vi "TX-SIS-BPCS-Modbus.vi"() -> ()   [LabVIEW 2018]
uses:
  <vilib>/Platform/TimedLoop/XDataNode/timing_clust.ctl
  <vilib>/Platform/TimedLoop/XDataNode/nitl_modes.ctl
  <vilib>/Platform/TimedLoop/XDataNode/wakeup.ctl
  <vilib>/Modbus/slave/Create Slave Instance (TCP).vi
  Global Variables.vi
  <vilib>/Modbus/slave/Modbus Slave.lvclass
  <vilib>/Platform/TimedLoop/XDataNode/XDataNode.xnode
  <vilib>/Platform/TimedLoop/XDataNode/XDNodeRunTimeDep.lvlib
panel:
  out "TX-SIS-BPCS-Array":bool[](array[boolean])
  in  "stop":bool
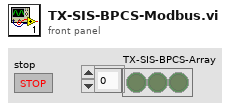
[diagram p1: front panel]
types:
  T1 = typedef "XDNodeRunTimeDep.lvlib/timing_clust.ctl" = cluster{"Expected End [f-1]":u64, "Actual End [f-1]":u64, "Finished Late? [f-1]":bool, "Expected End [i-1]":u64, "Actual End [i-1]":u64, "Finished Late? [i-1]":bool, "Expected Start [i]":u64, "Actual Start [i]":u64, "Expected Start [f]":u64, "Actual Start [f]":u64, "Source Name":string, "Structure Name":string, "Period":i64, "Deadline":i64, "Offset":i64, "Start":i64, "Priority":i32, "Timeout":i32, "Mode":T2, "Wakeup Reason":T3, "Error":errorcluster, "Source Type":string, "Secondary Source Type":string, "Global End Time":u64, "Global Start Time":u64, "Frame Duration":u64, "Iteration Duration":u64, "Assigned CPU":i32, "I/O Scan Engine Mode":u32}
  T2 = typedef "XDNodeRunTimeDep.lvlib/nitl_modes.ctl" = enum32{"No Change", "Process missed periods, maintain original phase", "Discard missed periods, maintain original phase", "Process missed periods, ignore original phase", "Discard missed periods, ignore original phase"}
  T3 = typedef "XDNodeRunTimeDep.lvlib/wakeup.ctl" = enum32{"Normal", "Aborted", "Asynchronous wakeup", "Timing source error", "Timed loop error", "Timeout"}
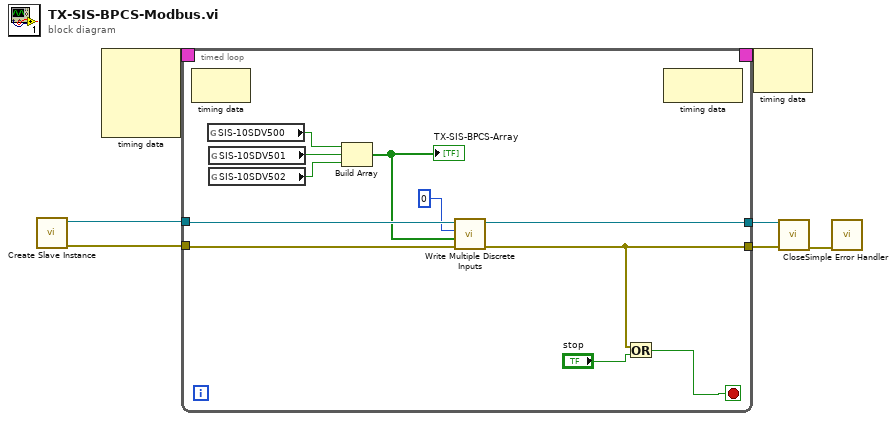
[diagram p0: block diagram]
diagram:
  n1 = call-poly <vilib>:"Create Slave Instance.vi"() -> ("error out"=w4:errorcluster, "TCP slave instance"=w5:refnum<class "Modbus Slave.lvclass">)  [unwired: 10 in]
  n2 = node-c288() -> (w7:T1)  [unwired: 4 in]
  n3 = timed-loop {
    timing: w7 -> [_]
    timing-out: [_] -> w6
    tunnel: w5 -> [w18]
    tunnel: w4 -> [w17]
    tunnel: [w11] -> w3
    tunnel: [w8] -> w2
    stop <- w10 stop-if-true
    n4 = node-c288() -> ()  [unwired: 1 in, 1 out]
    n5 = global read "Global Variables.vi" "SIS-10SDV500"() -> (w15:bool)
    n6 = global read "Global Variables.vi" "SIS-10SDV501"() -> (w13:bool)
    n7 = global read "Global Variables.vi" "SIS-10SDV502"() -> (w14:bool)
    n8 = Build Array(w15, w13, w14) -> (w12:bool[])
    "TX-SIS-BPCS-Array" <- w12
    n9 = call-dynamic "Write Multiple Discrete Inputs.vi"("error in (no error)"=w17, "discrete input values"=w12, "starting address"=u16 0, "Modbus slave in"=w18) -> ("error out"=w8:errorcluster, "Modbus slave out"=w11:refnum<class "Modbus Slave.lvclass">)  [unwired: 6 in]
    n10 = Or(x=w8, y="stop") -> (x .or. y?=w10:bool)
    n11 = node-c288() -> ()  [unwired: 1 in, 1 out]
  }
  n12 = node-c288(w6) -> ()  [unwired: 1 out]
  n13 = call-dynamic "Close.vi"("error in (no error)"=w2, "Modbus slave in"=w3) -> ("error out"=w1:errorcluster)  [unwired: 9 in]
  n14 = call <vilib>:"Simple Error Handler.vi"("error in (no error)"=w1) -> ()  [unwired: 4 in, 5 out]
